vi "Update Control Ref.vi"(8 "error in (no error)":errorcluster, 10 "Ctl Refnum":refnum<vi>, 11 "ElementEditorPanel in":refnum<class "ElementEditorPanel.lvclass">) -> (0 "error out":errorcluster, 3 "ElementEditorPanel out":refnum<class "ElementEditorPanel.lvclass">)   [LabVIEW 2020, in "VolatusGUIEditorCore.lvlib" / "ElementEditorPanel.lvclass"]
uses:
  ElementEditorPanel.lvclass
  ElementEditorPanel.lvclass/ElementEditorPanel.ctl
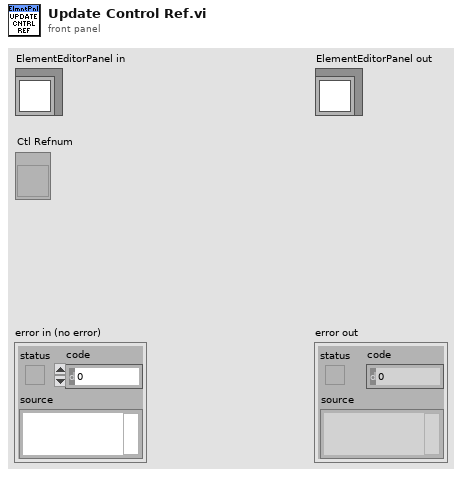
[diagram p1: front panel]
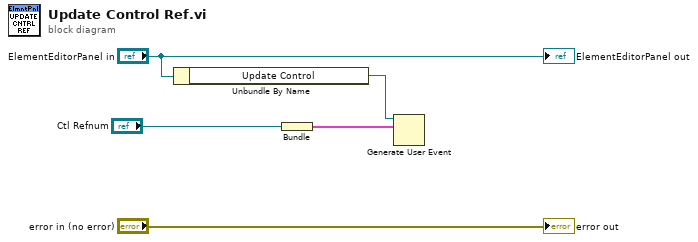
[diagram p0: block diagram]
diagram:
  n1 = Unbundle By Name("ElementEditorPanel in") -> ("Update Control"=w3:refnum<user-event>)
  n2 = Bundle("Ctl Refnum"="Ctl Refnum") -> (w1:cluster{"Ctl Refnum":refnum<vi>})  [unwired: 1 in]
  n3 = Generate User Event(user event=w3, event data cluster=w1) -> ()  [unwired: 2 in, 2 out]
  "error out" <- "error in (no error)"
  "ElementEditorPanel out" <- "ElementEditorPanel in"
